vi "BIMS_Collector Globals.vi"() -> ()   [LabVIEW 2015]
panel:
  in  "screenTasks":T1
  in  "LayerStitchTypeRefs":refnum<vi>[](array[refnum])
  in  "ScreensCntrIDs":T2
  in  "SampleAttribs":T3(array[cluster])
  in  "LayerSpecs":T4(array[cluster])
  in  "SampleStyles":refnum<vi>[](array[refnum])
  in  "Mfrs":refnum<vi>[](array[refnum])
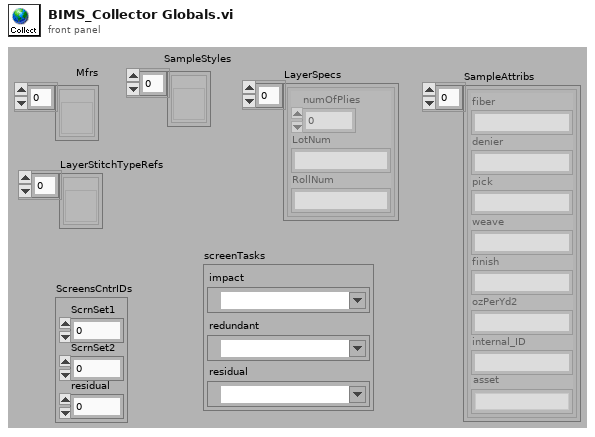
[diagram p1: front panel]
types:
  T1 = cluster{"impact":refnum<k21>, "redundant":refnum<k21>, "residual":refnum<k21>}
  T2 = cluster{"ScrnSet1":u32, "ScrnSet2":u32, "residual":u32}
  T3 = cluster{"fiber":string, "denier":string, "pick":string, "weave":string, "finish":string, "ozPerYd2":string, "internal_ID":string, "asset":string}[]
  T4 = cluster{"numOfPlies":i32, "LotNum":string, "RollNum":string}[]
diagram:
